vi "Main.vi"() -> ()   [LabVIEW 2016]
panel:
  out "Waveform Chart":dbl(graph)
  out "number (0 to 1)":dbl
  in  "Stop":bool
  # "Umsch. + TAB  Multitool"
  # "STRG + E"
  # "STRG + Leer"
  # "STRG + R"
  # "STRG + B"
  # "STRG +"
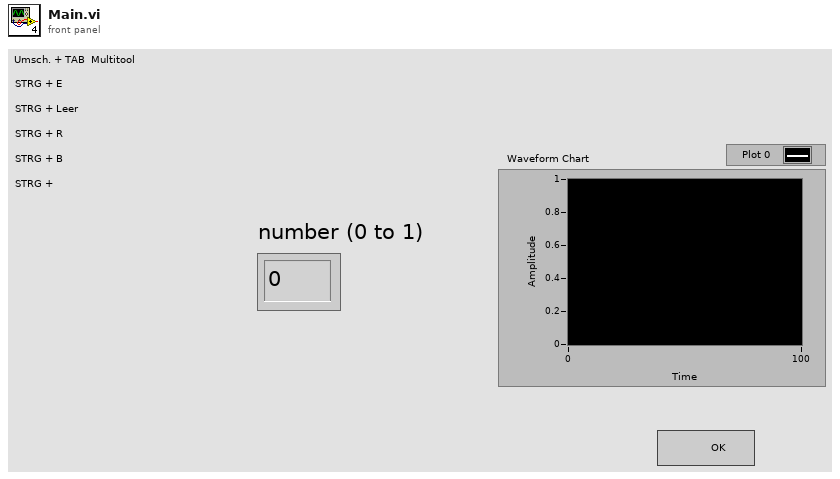
[diagram p1: front panel]
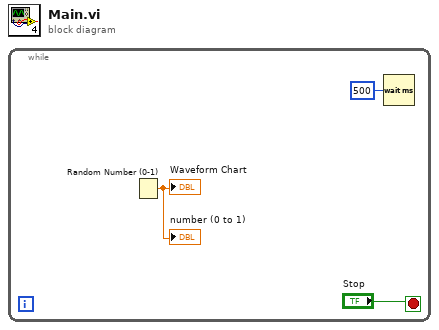
[diagram p0: block diagram]
diagram:
  n1 = while {
    stop <- "Stop" stop-if-true
    n2 = Random Number (0-1)() -> (number: 0 to 1=→"number (0 to 1)" →"Waveform Chart":dbl)
    n3 = Wait (ms)(milliseconds to wait=u32 500) -> ()  [unwired: 1 out]
  }
